vi "Threshold Color.vi"(2 "error in (no error)":errorcluster, 3 "Range":cluster{"Lower value":sgl, "Upper value":sgl}={"Lower value"=128.0, "Upper value"=255.0} {"Upper value" format="%.2f"; "Lower value" format="%.2f"}, 4 "Image Dst":T1, 5 "Image Src":T1) -> (0 "error out":errorcluster, 1 "Image Dst Out":T1)   [LabVIEW 2009, in "ImageProcessing.lvlib"]
doc: "Thresholds a grayscaled image and does som clean up"
uses:
  ImageProcessing.lvlib
  <vilib>/vision/Image Controls.llb/IMAQ Image.ctl
  <vilib>/vision/NI_Vision_Development_Module.lvlib
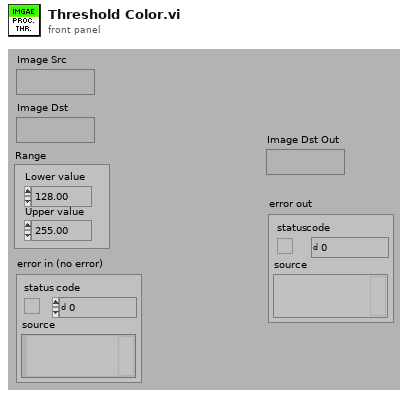
[diagram p1: front panel]
types:
  T1 = typedef "IMAQ Image.ctl" = refnum<image>
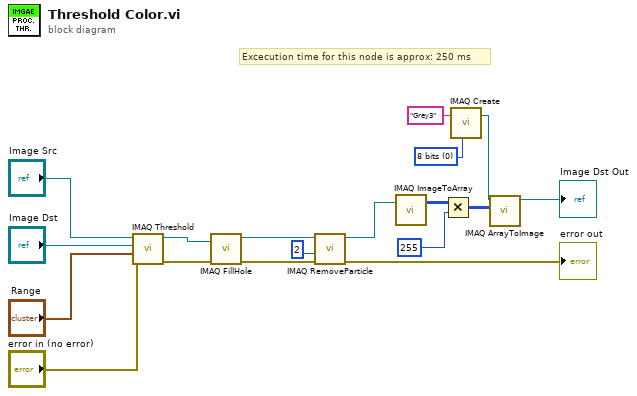
[diagram p0: block diagram]
diagram:
  w5 = u32 0 items=["8 bits", "16 bits", "Float", "Complex", "RGB", "HSL"] ("Image Type")
  # "Excecution time for this node is approx: 250 ms"
  n1 = call "IMAQ Threshold"("error in (no error)"="error in (no error)", "Range"="Range", "Image Dst"="Image Dst", "Image Src"="Image Src") -> ("error out"=w15:errorcluster, "Image Dst Out"=w11:T1)  [unwired: 6 in]
  n2 = call "IMAQ FillHole"("error in (no error)"=w15, "Image Src"=w11) -> ("error out"=w14:errorcluster, "Image Dst Out"=w10:T1)  [unwired: 2 in, 2 out]
  n3 = call "IMAQ RemoveParticle"("error in (no error)"=w14, "Number of Erosion"=2, "Image Src"=w10) -> ("error out"=→"error out":errorcluster, "Image Dst Out"=w3:T1)  [unwired: 4 in, 3 out]
  n4 = call "IMAQ ImageToArray"("Image"=w3) -> ("Image Pixels (U8)"=w9:u8[][])  [unwired: 3 in, 4 out]
  n5 = Multiply(x=w9, y=255) -> (x*y=w7:i32[][])
  n6 = call "IMAQ Create"("Image Name"="Grey3", "Image Type"=w5) -> ("New Image"=w4:T1)  [unwired: 2 in, 2 out]
  n7 = call "IMAQ ArrayToImage"("Image Pixels (U8)"=w7, "Image"=w4) -> ("Image Out"=→"Image Dst Out":T1)  [unwired: 8 in, 1 out]
